vi "Output Speed.vi"(8 "Iteration":i32, 9 "Time Delay":i32, 10 "Feedback":dbl, 11 "In":dbl) -> (0 "Iteration Out":i32, 3 "Out":dbl)   [LabVIEW 2012]
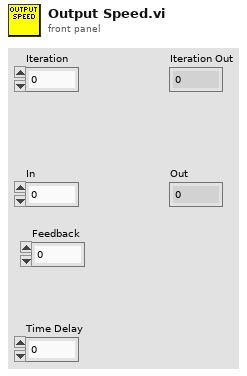
[diagram p1: front panel]
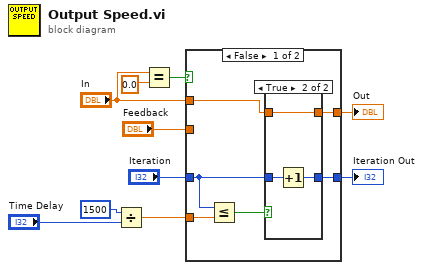
[diagram p0: block diagram]
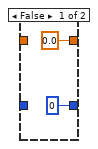
[diagram p2: hidden frame]
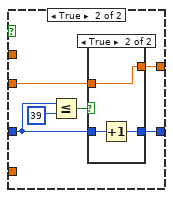
[diagram p3: hidden frame]
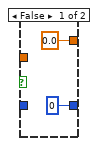
[diagram p4: hidden frame]
diagram:
  n1 = Divide(x=1500, y="Time Delay") -> (x/y=w1:dbl)
  n2 = Equal?(x="In", y=0.0) -> (x = y?=w8:bool)
  n3 = case shown="False" w8 {
    tunnel: "In" -> [w13 _]
    tunnel: "Iteration" -> [w15 w24]
    tunnel: [w14 w22] -> w9
    tunnel: [w12 w25] -> w5
    tunnel: "Feedback" -> [_ w23]
    tunnel: w1 -> [w11 _]
    frame False {
      n4 = Less Or Equal?(x=w15, y=w11) -> (x <= y?=w16:bool)
      n5 = case shown="True" w16 {
        tunnel: w15 -> [_ w21]
        tunnel: [0 w20] -> w12
        tunnel: [0.0 ("In") w19] -> w14
        tunnel: w13 -> [_ w19]
        frame False {
        }
        frame True {
          n6 = Increment(x=w21) -> (x+1=w20:i32)
        }
      }
    }
    frame True {
      n7 = Less Or Equal?(x=w24, y=39) -> (x <= y?=w27:bool)
      n8 = case shown="True" w27 {
        tunnel: w24 -> [_ w32]
        tunnel: [0 w31] -> w25
        tunnel: [0.0 ("In") w30] -> w22
        tunnel: w23 -> [_ w30]
        frame False {
        }
        frame True {
          n9 = Increment(x=w32) -> (x+1=w31:i32)
        }
      }
    }
  }
  "Out" <- w9
  "Iteration Out" <- w5
